vi "电流值.vi"() -> ()   [LabVIEW 2021]
panel:
  out "电源电流":dbl format="%#_6f A"
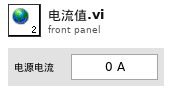
[diagram p1: front panel]
diagram:
